vi "Add APU.vi"(8 "error in (no error)":errorcluster, 10 "APU Settings":T1 {"des accel" min=0.0 format="%#_p"}, 11 "EST Custom Device in":refnum<k24>) -> (0 "error out":errorcluster, 2 "APU":refnum<k24>, 3 "EST Custom Device out":refnum<k24>)   [LabVIEW 2015, in "Engine Simulation Toolkit Scripting API.lvlib"]
uses:
  Engine Simulation Toolkit Scripting API.lvlib
  NationalInstruments.VeriStand.SystemDefinitionAPI
  APU Settings.ctl
  System Explorer/Engine Simulation Toolkit System Explorer.lvlib
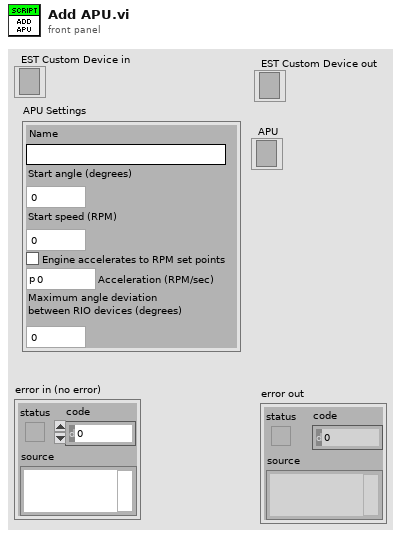
[diagram p1: front panel]
types:
  T1 = typedef "Engine Simulation Toolkit Scripting API.lvlib/APU Settings.ctl" = cluster{"Name":string, "Start angle (degrees)":dbl, "des speed":dbl, "Acceleration":bool, "des accel":dbl, "Maximum angle deviation\nbetween RIO devices (degrees)":dbl}
  T2 = typedef "Custom Device API.lvlib/Custom Device Item Ref.ctl" = u64
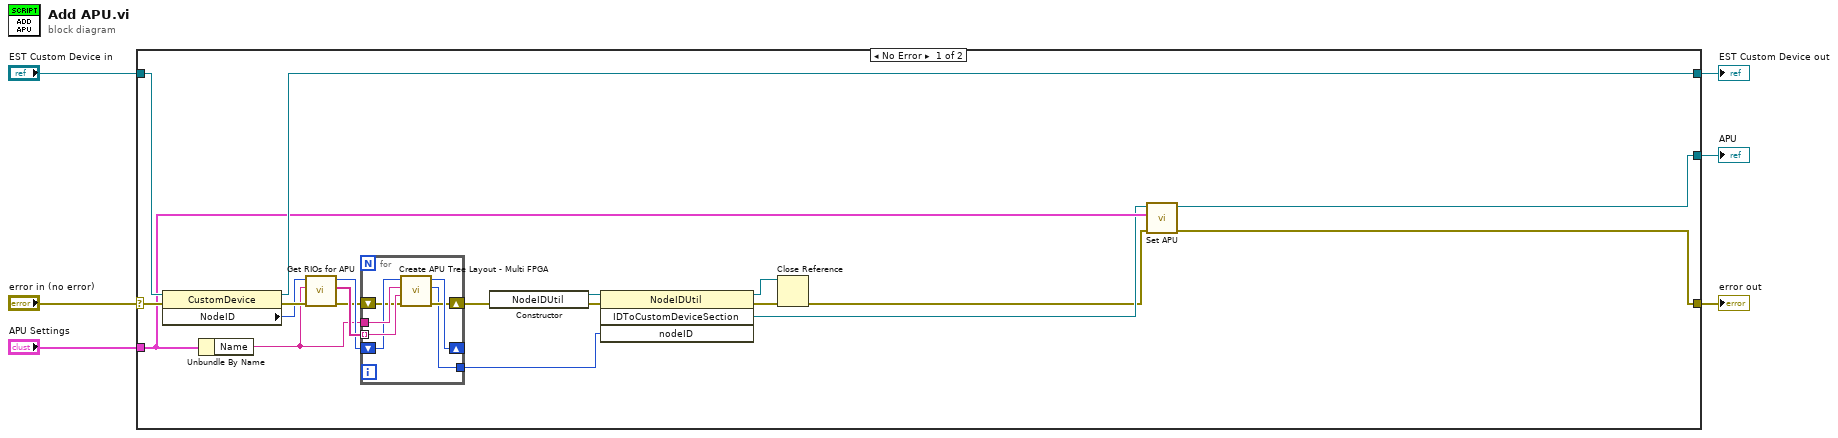
[diagram p0: block diagram]
diagram:
  n1 = case shown="No Error" "error in (no error)" {
    selector: "error in (no error)" -> [w25 w35]
    tunnel: [w9 w35] -> w6
    tunnel: "EST Custom Device in" -> [w26 w34]
    tunnel: [w24 w34] -> w3
    tunnel: "APU Settings" -> [w18 _]
    tunnel: [w10 _] -> w1
    frame No Error {
      n2 = property class="CustomDevice"(reference=w26, error in=w25) -> (reference out=w24:refnum<k24>, error out=w23:errorcluster, "NodeID"=w22:u64)
      n3 = Unbundle By Name(w18) -> ("Name"=w17:string)
      n4 = call "Get RIOs for APU.vi"("error in (no error)"=w23, "APU name"=w17, "Item Ref in"=w22) -> ("error out"=w19:errorcluster, "RIO Addresses"=w21:string[], "Item Ref out"=w20:T2)  [unwired: 6 in]
      n5 = for {
        tunnel: w21 -> [w33] mode=indexing
        tunnel: w17 -> [w32]
        shift-right: [w28] -> w8
        shift-left: w19 -> [w30]
        shift-right: [w29] -> _
        shift-left: w20 -> [w31]
        tunnel: [w27] -> w12
        n6 = call "Create APU Tree Layout - Multi FPGA.vi"("error in (no error)"=w30, "rio name"=w33, "engine name"=w32, "Section Ptr"=w31) -> ("error out"=w28:errorcluster, "APU ref"=w27:T2, "Section Ptr dup"=w29:T2)  [unwired: 5 in]
      }
      n7 = constructor class="NodeIDUtil"(error in=w8) -> (reference out=w15:refnum<k24>, error out=w16:errorcluster)  [unwired: 2 in, 1 out]
      n8 = invoke class="NodeIDUtil" method="IDToCustomDeviceSection"(reference=w15, error in=w16, "nodeID"=w12) -> (reference out=w14:refnum<k24>, error out=w13:errorcluster, "IDToCustomDeviceSection"=w11:refnum<k24>)  [unwired: 1 in, 1 out]
      n9 = Close Reference(reference=w14, error in (no error)=w13) -> (error out=w7:errorcluster)
      n10 = call "Set APU.vi"("error in (no error)"=w7, "APU Settings"=w18, "APU in"=w11) -> ("error out"=w9:errorcluster, "APU out"=w10:refnum<k24>)  [unwired: 7 in]
    }
    frame Error {
    }
  }
  "EST Custom Device out" <- w3
  "error out" <- w6
  "APU" <- w1
